vi "GetVarParRowCol.vi"(8 "ErrorIn(No Error)":errorcluster caption="entrée d'erreur (pas d'erreur)", 10 "VarPar":string, 11 "VarParams":string[][](array[string])) -> (0 "sortie d'erreur":errorcluster, 2 "Col":i32, 3 "Line":i32)   [LabVIEW 2019]
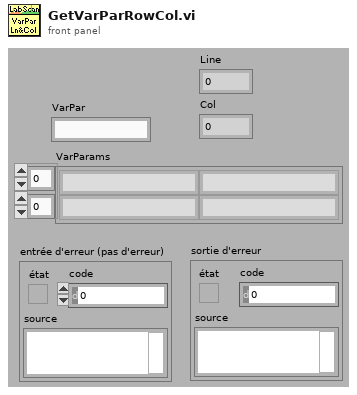
[diagram p1: front panel]
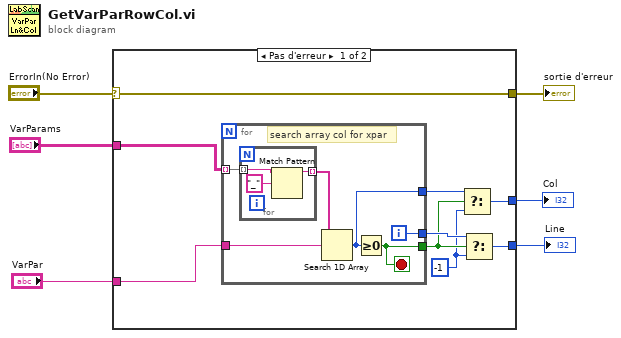
[diagram p0: block diagram]
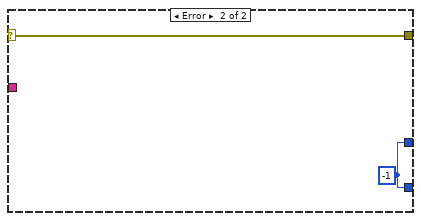
[diagram p2: hidden frame]
diagram:
  n1 = case shown="Pas d'erreur" "ErrorIn(No Error)" {
    selector: "ErrorIn(No Error)" -> [w12 w26]
    tunnel: [w12 w26] -> w5
    tunnel: "VarPar" -> [w15 _]
    tunnel: "VarParams" -> [w7 _]
    tunnel: [w13 w25] -> w1
    tunnel: [w8 w25] -> w2
    frame No Error {
      w9 = -1 ("cas faux")
      n2 = for {
        tunnel: w7 -> [w18] mode=indexing
        tunnel: w15 -> [w21]
        tunnel: [w20] -> w14
        tunnel: [w19] -> w10
        tunnel: [w16] -> w11
        i -> [w20]
        stop <- w19 stop-if-true
        # "search array col for xpar"
        n3 = for {
          tunnel: w18 -> [w24] mode=indexing
          tunnel: [w23] -> w17 mode=indexing
          n4 = Match Pattern(string=w24, regular expression="_" ("expression régulière")) -> (before substring=w23:string)  [unwired: 1 in, 3 out]
        }
        n5 = Search 1D Array(1D array=w17, element=w21) -> (index of element=w16:i32)  [unwired: 1 in]
        n6 = Greater Or Equal To 0?(x=w16) -> (x >= 0?=w19:bool)
      }
      n7 = Select(t=w11, s=w10, f=w9) -> (s? t:f=w8:i32)
      n8 = Select(t=w14, s=w10, f=w9) -> (s? t:f=w13:i32)
    }
    frame Error {
      w25 = -1
    }
  }
  "sortie d'erreur" <- w5
  "Col" <- w2
  "Line" <- w1
